vi "Read configuration.vi"(8 "error in (no error)":errorcluster, 11 "Fgen Instrument":refnum<class "Fgen Instrument.lvclass">) -> (0 "error out":errorcluster, 2 "configuration":refnum<class "CEF_serializable configuration.lvclass">, 3 "Fgen Instrument out":refnum<class "Fgen Instrument.lvclass">)   [LabVIEW 2025, in "Fgen.lvlib" / "Fgen Instrument.lvclass"]
uses:
  Fgen Instrument.lvclass
  Users/Public/Documents/Sandia National Labs/TSS Plugin/CEF.lvlibp/serializable configuration/CEF_serializable configuration.lvclass
  Fgen Instrument.lvclass/Fgen Instrument.ctl
  Fgen configuration/Fgen configuration.lvclass
  C:/Users/Public/Documents/Sandia National Labs/TSS Plugin/CEF.lvlibp/serializable configuration/CEF_serializable configuration.lvclass
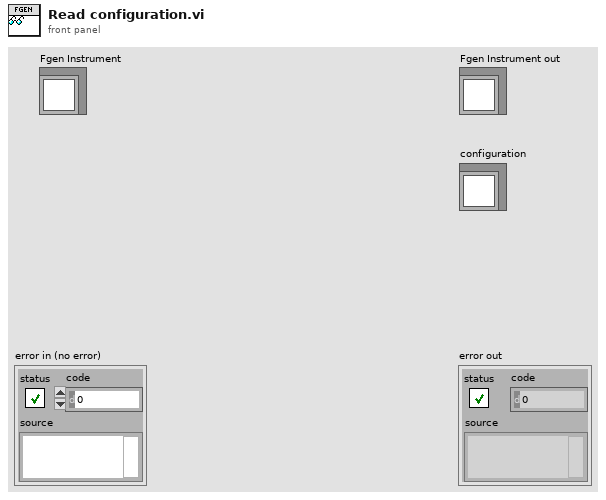
[diagram p1: front panel]
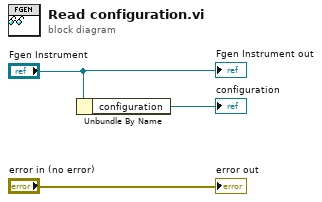
[diagram p0: block diagram]
diagram:
  n1 = Unbundle By Name("Fgen Instrument") -> ("configuration"=→"configuration":refnum<class "Fgen configuration.lvclass">)
  "error out" <- "error in (no error)"
  "Fgen Instrument out" <- "Fgen Instrument"
